vi "FileName.vi"() -> (0 "dup directory path":path, 1 "String":string)   [LabVIEW 2015]
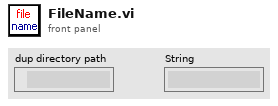
[diagram p1: front panel]
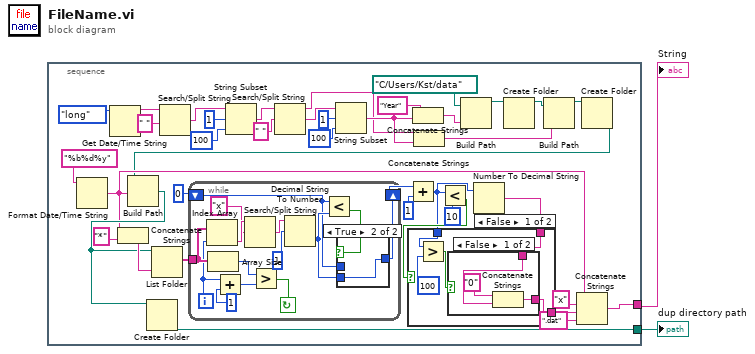
[diagram p0: block diagram]
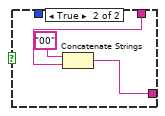
[diagram p4: hidden frame]
diagram:
  n1 = stacked-sequence {
    tunnel: [w5] -> w2
    tunnel: [w4] -> w1
    frame #0 {
      n2 = Format Date/Time String(time format string (%c)="%b%d%y") -> (date/time string=w10:string)  [unwired: 2 in]
      n3 = Get Date/Time String(date format (0)=enum16{"short", "long", "abbreviated"}."long") -> (date string=w26:string)  [unwired: 2 in, 1 out]
      n4 = Concatenate Strings(w10, "*") -> (w34:string)
      n5 = Search/Split String(string=w26, search string/char (-)=" ") -> (match + rest of string=w24:string)  [unwired: 1 in, 2 out]
      n6 = String Subset(string=w24, offset (0)=1, length (rest)=100 ("length (rest)")) -> (substring=w17:string)
      n7 = Search/Split String(string=w17, search string/char (-)=" ") -> (substring before match=w13:string, match + rest of string=w18:string)  [unwired: 1 in, 1 out]
      n8 = String Subset(string=w18, offset (0)=1, length (rest)=100 ("length (rest)")) -> (substring=w14:string)
      n9 = Concatenate Strings("Year" ("Substring"), w14) -> (w15:string)
      n10 = Concatenate Strings(w13, w14) -> (w12:string)
      n11 = Build Path(base path=path "C:/Users/Kst/data", name or relative path=w15) -> (appended path=w9:path)
      n12 = Create Folder(path (use dialog)=w9) -> (created path=w8:path)  [unwired: 2 in, 2 out]
      n13 = Build Path(base path=w8, name or relative path=w12) -> (appended path=w7:path)
      n14 = Create Folder(path (use dialog)=w7) -> (created path=w6:path)  [unwired: 2 in, 2 out]
      n15 = Build Path(base path=w6, name or relative path=w10) -> (appended path=w11:path)
      n16 = Create Folder(path (use dialog)=w11) -> (created path=w5:path)  [unwired: 2 in, 2 out]
      n17 = List Folder(path=w11, pattern=w34) -> (filenames=w35:string[])  [unwired: 2 in, 3 out]
      n18 = while {
        shift-left: 0 -> [w48]
        shift-right: [w47] -> w37
        tunnel: w35 -> [w44]
        i -> [w43]
        stop <- w53 continue-if-true
        n19 = Index Array(array=w44, index=w43) -> (element=w52:string)
        n20 = Array Size(array=w44) -> (size(s)=w55:i32)
        n21 = Add(x=w43, y=1) -> (x+y=w42:i32)
        n22 = Search/Split String(string=w52, search string/char (-)="x") -> (match + rest of string=w46:string)  [unwired: 1 in, 2 out]
        n23 = Greater?(x=w55, y=w42) -> (0:w53:bool)
        n24 = Decimal String To Number(string=w46, offset=1) -> (number=w49:i32)  [unwired: 1 in, 1 out]
        n25 = Less?(x=w48, y=w49) -> (x < y?=w50:bool)
        n26 = case shown="True" w50 {
          tunnel: w49 -> [_ w57]
          tunnel: w48 -> [w56 _]
          tunnel: [w56 w57] -> w47
          frame False {
          }
          frame True {
          }
        }
      }
      n27 = Add(x=w37, y=1) -> (x+y=w29:i32)
      n28 = Less?(x=w29, y=10) -> (x < y?=w31:bool)
      n29 = Number To Decimal String(number=w29) -> (decimal integer string=w30:string)  [unwired: 1 in]
      n30 = case shown="False" w31 {
        tunnel: w30 -> [w59 w69]
        tunnel: [w58 w67] -> w28
        tunnel: w29 -> [w61 _]
        frame False {
          n31 = Greater?(x=w61, y=100) -> (0:w60:bool)
          n32 = case shown="False" w60 {
            tunnel: w59 -> [w64 w66]
            tunnel: [w63 w66] -> w58
            frame False {
              n33 = Concatenate Strings("0", w64) -> (w63:string)
            }
            frame True {
            }
          }
        }
        frame True {
          n34 = Concatenate Strings("00", w69) -> (w67:string)
        }
      }
      n35 = Concatenate Strings(w10, "x", w28, ".dat" ("Substring")) -> (w4:string)
    }
  }
  "dup directory path" <- w2
  "String" <- w1
